vi "2Channel_ControlFiles.vi"() -> ()   [LabVIEW 2013]
uses:
  <vilib>/DAQmx/write.llb/DAQmx Write (Analog 2D DBL NChan NSamp).vi
  <vilib>/Utility/file.llb/Read From Spreadsheet File (DBL).vi
  <vilib>/DAQmx/create/channels.llb/DAQmx Create Channel (AO-Voltage-Basic).vi
  <vilib>/DAQmx/configure/timing.llb/DAQmx Timing (Sample Clock).vi
  <vilib>/DAQmx/miscellaneous.llb/DAQmx Fill In Error Info.vi
  <resource>/objmgr/daqmx.rc
panel:
  out "Control Graph":T1(graph)
  out "Actual Clock Rate":dbl
  out "Total Samples":i32
  out "Total Time [minutes]":dbl format="%.2f"
  in  "Update Rate [Hz]":dbl=10.0
  # "Instructions:\n\n1) Set the update rate in the VI\n2) Click the run arrow\n3) Select the desired control file\n4) Prepare your experiment and lock the piston\n5) Start the file and a stopwatch\n6) Switch the control signal in and zero the pointer\n7) Unlock the piston\n\nVersion 1.0.1\nJ.R. Leeman\nkd5wxb@gmail.com"
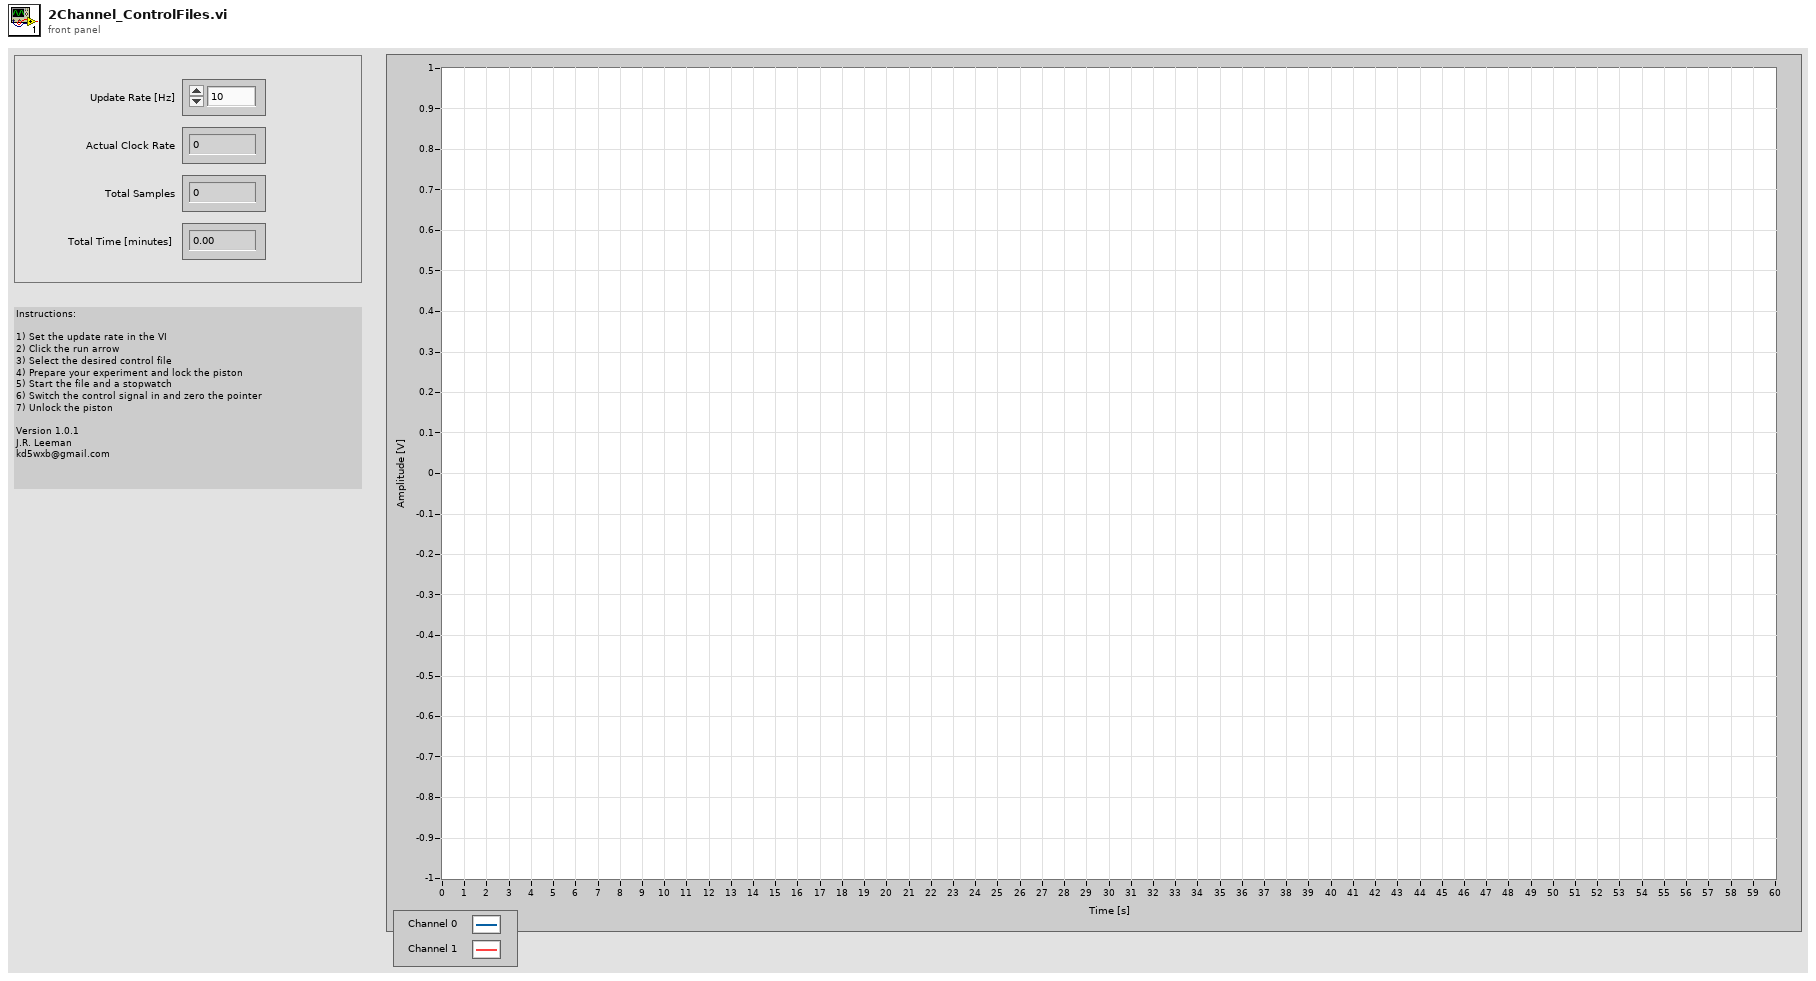
[diagram p1: front panel]
types:
  T1 = cluster{"minimum value":dbl, dbl, "all rows":dbl[][]}
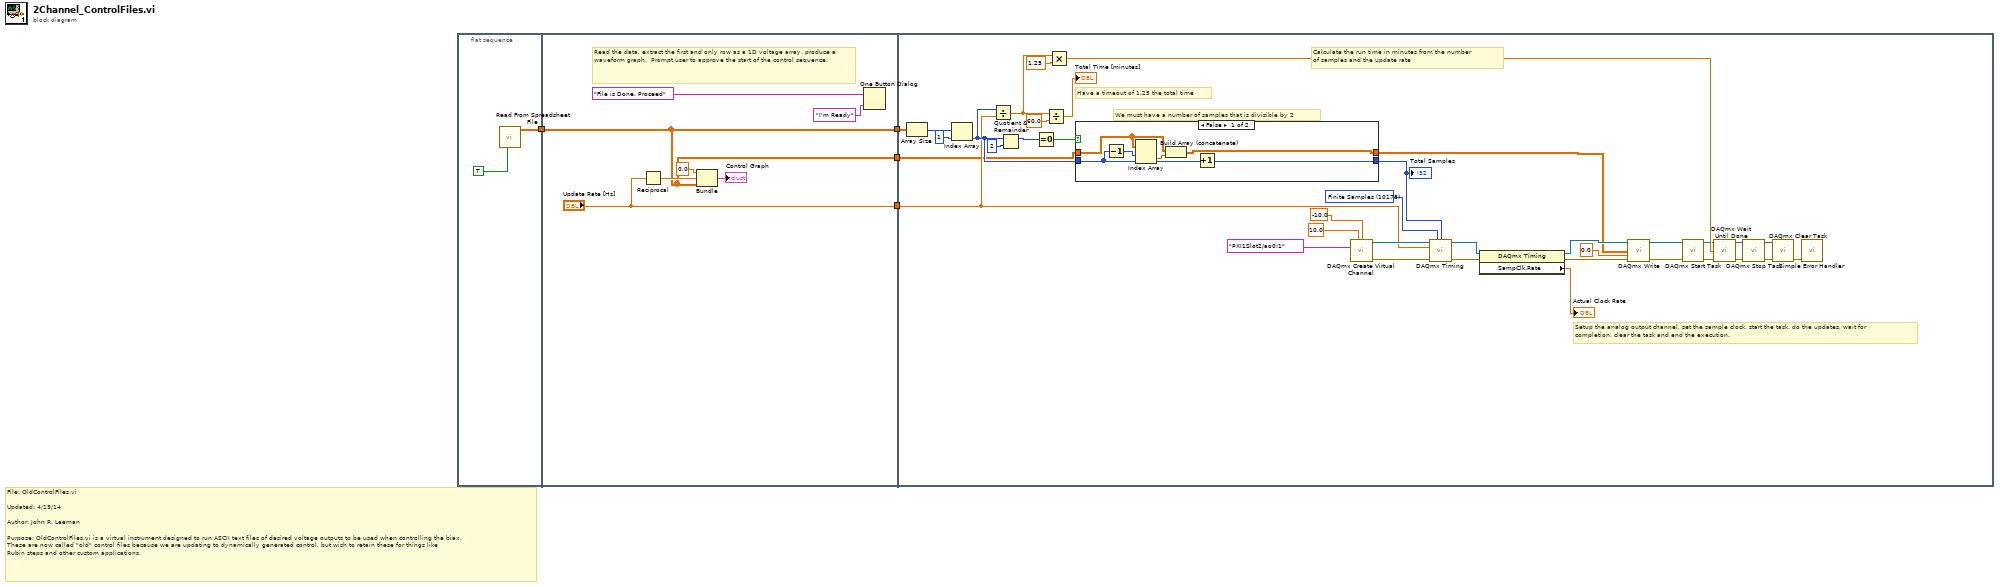
[diagram p0: block diagram]
diagram:
  # "File: OldControlFiles.vi\n\nUpdated: 4/19/14\n\nAuthor: John R. Leeman\n\nPurpose: OldControlFiles.vi is a virtual instrument designed to run ASCII text files of desired voltage outputs to be used when controlling the biax.\nThese are now called \"old\" control files because we are updating to dynamically generated control, but wish to retain these for things like\nRubin steps and other custom applications."
  n1 = flat-sequence {
    tunnel: [w5] -> w4
    tunnel: w4 -> [w7]
    tunnel: [w7] -> w3
    tunnel: ["Update Rate [Hz]"] -> w2
    tunnel: [w7] -> w1
    tunnel: w3 -> [w33]
    tunnel: w2 -> [w16]
    tunnel: w1 -> [w15]
    frame #0 {
      n2 = call-poly <vilib>:"Read From Spreadsheet File.vi"("transpose (no:F)"=TRUE) -> ("all rows"=w5:dbl[][])  [unwired: 6 in, 4 out]
    }
    frame #1 {
      # "Read the data, extract the first and only row as a 1D voltage array, produce a waveform graph.  Prompt user to approve the start of the control sequence."
      n3 = Reciprocal(x="Update Rate [Hz]") -> (1/x=w11:dbl)
      n4 = Bundle("minimum value"=0.0, w11, "all rows"=w7) -> (→"Control Graph":T1)  [unwired: 1 in]
      n5 = One Button Dialog(message="File is Done. Proceed", button name ("OK")="I'm Ready") -> ()  [unwired: 1 out]
    }
    frame #2 {
      w46 = 10178 items=["Finite Samples"=10178, "Continuous Samples"=10123, "Hardware Timed Single Point"=12522] ("sample mode")
      # "Have a timeout of 1.25 the total time"
      # "We must have a number of samples that is divisible by 2"
      # "Setup the analog output channel, set the sample clock, start the task, do the updates, wait for \ncompletion, clear the task and end the execution."
      # "Calculate the run time in minutes from the number \nof samples and the update rate"
      n6 = Array Size(array=w33) -> (size(s)=w45:i32[])
      n7 = Index Array(array=w45, index=1) -> (element=w18:i32)
      n8 = Divide(x=w18, y=w16) -> (x/y=w41:dbl)
      n9 = Quotient & Remainder(x=w18, y=2) -> (x-y*floor(x/y)=w20:i32)  [unwired: 1 out]
      n10 = Equal To 0?(x=w20) -> (x = 0?=w19:bool)
      n11 = Divide(x=w41, y=60.0) -> (x/y=→"Total Time [minutes]":dbl)
      n12 = Multiply(x=w41, y=1.25) -> (x*y=w40:dbl)
      n13 = case shown="False" w19 {
        tunnel: w15 -> [w54 w58]
        tunnel: [w52 w58] -> w14
        tunnel: [w56 w57] -> w17
        tunnel: w18 -> [w55 w57]
        frame False {
          n14 = Decrement(x=w55) -> (x-1=w51:i32)
          n15 = Index Array(array=w54, index (row)=w51) -> (element=w53:dbl[])  [unwired: 1 in]
          n16 = Build Array (concatenate)(w54, w53) -> (w52:dbl[][])
          n17 = Increment(x=w55) -> (x+1=w56:i32)
        }
        frame True {
        }
      }
      "Total Samples" <- w17
      n18 = call-poly <vilib>:"DAQmx Create Virtual Channel.vi"("maximum value"=10.0, "minimum value"=-10.0, "physical channels"=tag "PXI1Slot2/ao0:1") -> ("task out"=w50:refnum<k21>, "error out"=w49:errorcluster)  [unwired: 11 in]
      n19 = call-poly <vilib>:"DAQmx Timing.vi"("task/channels in"=w50, "sample mode"=w46, "samples per channel"=w17, "rate"=w16, "error in"=w49) -> ("task out"=w32:refnum<k21>, "error out"=w29:errorcluster)  [unwired: 9 in]
      n20 = property class="DAQmx Timing"(reference=w32, error in=w29) -> (reference out=w27:refnum<k21>, error out=w26:errorcluster, "SampClk.Rate"=→"Actual Clock Rate":dbl)
      n21 = call-poly <vilib>:"DAQmx Write.vi"("task/channels in"=w27, "data"=w14, "timeout"=0.0, "error in"=w26) -> ("task out"=w25:refnum<k21>, "error out"=w22:errorcluster)  [unwired: 9 in, 1 out]
      n22 = call <vilib>:"DAQmx Start Task.vi"("task/channels in"=w25, "error in"=w22) -> ("task out"=w24:refnum<k21>, "error out"=w23:errorcluster)  [unwired: 12 in]
      n23 = call <vilib>:"DAQmx Wait Until Done.vi"("task/channels in"=w24, "timeout (sec)"=w40, "error in"=w23) -> ("task out"=w31:refnum<k21>, "error out"=w36:errorcluster)  [unwired: 11 in]
      n24 = call <vilib>:"DAQmx Stop Task.vi"("task/channels in"=w31, "error in"=w36) -> ("task out"=w30:refnum<k21>, "error out"=w37:errorcluster)  [unwired: 12 in]
      n25 = call <vilib>:"DAQmx Clear Task.vi"("task in"=w30, "error in"=w37) -> ("error out"=w48:errorcluster)  [unwired: 13 in]
      n26 = call <vilib>:"Simple Error Handler.vi"("error in (no error)"=w48) -> ()  [unwired: 4 in, 5 out]
    }
  }
